vi "ConfigureOutputTrigger.vi"(0 "object in":refnum<class "Hamamatsu.lvclass">, 2 "Trigger Output Settins":T1={"Output Trigger Type"={"Mode"=1, "Polarity"=1}, "Programmable Options"={"Width"=0.003, "Delay"=0.0, "Source"=2}, "Port"=1} {"Output Trigger Type"."Mode" items=["Low"=1, "Global Exposure"=2, "Programmable"=3, "Trigger Ready"=4, "High"=5]; "Output Trigger Type"."Polarity" items=["Negative"=1, "Positive"=2]; "Programmable Options"."Source" items=["Exposure"=1, "Readout End"=2, "V Sync"=3, "H Sync"=4, "Trigger"=6]}, 5 "error in (no error)":errorcluster) -> (14 "object out":refnum<class "Hamamatsu.lvclass">, 19 "error out":errorcluster)   [LabVIEW 2023, in "Hamamatsu.lvclass"]
uses:
  Hamamatsu.lvclass
  Hamamatsu.lvclass/Hamamatsu.ctl
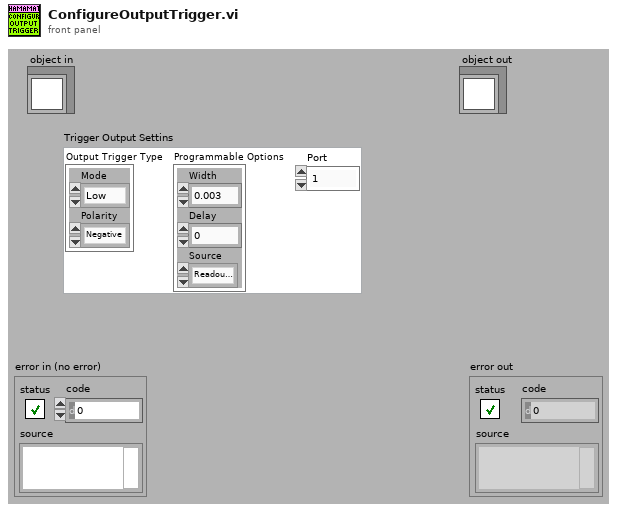
[diagram p1: front panel]
types:
  T1 = cluster{"Output Trigger Type":cluster{"Mode":u32, "Polarity":u32}, "Programmable Options":cluster{"Width":dbl, "Delay":dbl, "Source":u32}, "Port":i32}
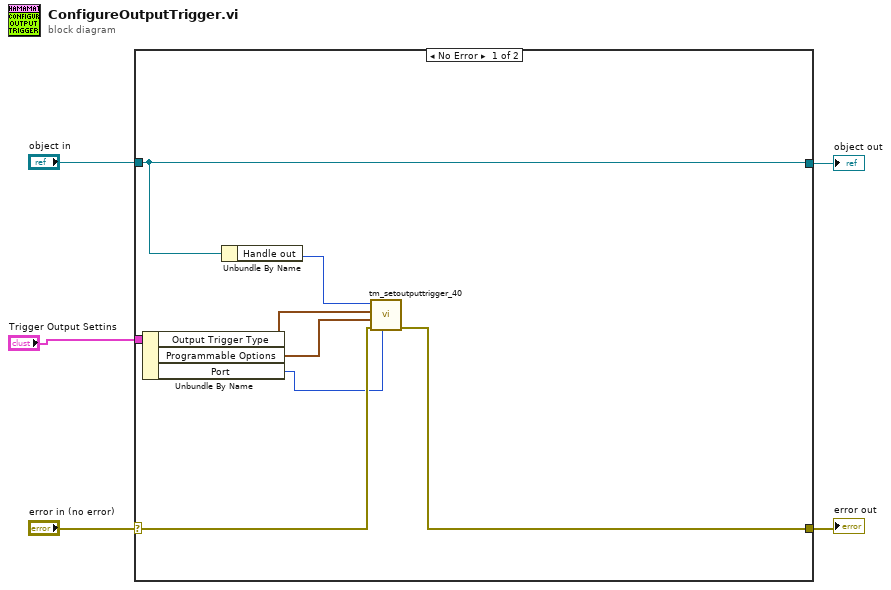
[diagram p0: block diagram]
diagram:
  n1 = case shown="No Error" "error in (no error)" {
    selector: "error in (no error)" -> [w11 w15]
    tunnel: [w10 w15] -> w4
    tunnel: [w13 w14] -> w2
    tunnel: "object in" -> [w13 w14]
    tunnel: "Trigger Output Settins" -> [w9 _]
    frame No Error {
      n2 = Unbundle By Name(w9) -> ("Output Trigger Type"=w8:cluster{"Mode":u32, "Polarity":u32}, "Programmable Options"=w7:cluster{"Width":dbl, "Delay":dbl, "Source":u32}, "Port"=w6:i32)
      n3 = Unbundle By Name(w13) -> ("Handle out"=w12:u32)
      n4 = call <userlib>:"tm_setoutputtrigger_40.vi"("Port"=w6, "error in (no error)"=w11, "Programmable Options"=w7, "Type"=w8, "Handle in"=w12) -> ("error out"=w10:errorcluster)  [unwired: 5 in, 1 out]
    }
    frame Error {
    }
  }
  "error out" <- w4
  "object out" <- w2
